vi "Notify Command Complete.vi"(0 "LVx.lvlib:LVx.lvclass":refnum<class "LVx.lvclass">, 11 "error in (no error)":errorcluster) -> (4 "LVx.lvclass out":refnum<class "LVx.lvclass">, 15 "error out":errorcluster)   [LabVIEW 2011, in "LVx.lvlib" / "LVx.lvclass"]
uses:
  LVx.lvclass
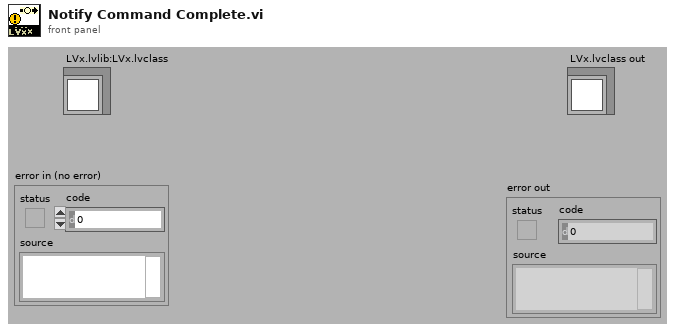
[diagram p1: front panel]
types:
  T1 = typedef "LVx.lvlib/LVx.lvclass/Typedef - LVx Response Notifier.ctl" = refnum<notifier>
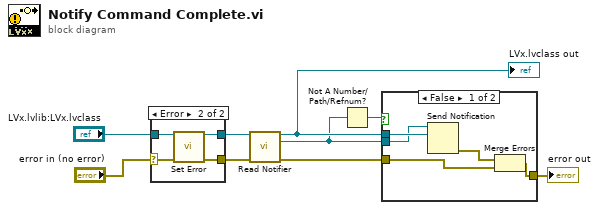
[diagram p0: block diagram]
diagram:
  n1 = case shown="Error" "error in (no error)" {
    selector: "error in (no error)" -> [w11 w12]
    tunnel: "LVx.lvlib:LVx.lvclass" -> [w10 w15]
    tunnel: [w11 w14] -> w7
    tunnel: [w10 w13] -> w5
    frame No Error {
    }
    frame Error {
      n2 = call "Set Error.vi"("LVx.lvlib:LVx.lvclass"=w15, "error in (no error)"=w12) -> ("LVx.lvlib:LVx.lvclass 2"=w13:refnum<class "LVx.lvclass">, "error out"=w14:errorcluster)  [unwired: 12 out]
    }
  }
  n3 = call "Read Notifier.vi"("LVx.lvclass in"=w5, "error in (no error)"=w7) -> ("LVx.lvclass out"=w4:refnum<class "LVx.lvclass">, "response notifier"=w3:T1, "error out"=w6:errorcluster)  [unwired: 11 out]
  "LVx.lvclass out" <- w4
  n4 = Not A Number/Path/Refnum?(number/path/refnum=w3) -> (NaN/Path/Refnum?=w2:bool)
  n5 = case shown="False" w2 {
    tunnel: [w20 w21] -> w8
    tunnel: w6 -> [w18 w21]
    tunnel: w4 -> [w17 _]
    tunnel: w3 -> [w16 _]
    frame False {
      n6 = Send Notification(notification=w17, notifier=w16) -> (error out=w19:errorcluster)  [unwired: 1 in, 1 out]
      n7 = Merge Errors(w19, w18) -> (w20:errorcluster)
    }
    frame True {
    }
  }
  "error out" <- w8
